vi "Photostimulation UI.vi"() -> ()   [LabVIEW 2012]
uses:
  GFG/GFGnumericGet.vi
  GFG/GFG library.lvlib
  <vilib>/vision/NI_Vision_Development_Module.lvlib
panel:
  out "deco string":string="Press and hold Ctrl to add multiple ROIs" caption="multiple points"
  in  "number of spots":dbl=5e-05 min=0.0 max=1.0 step=1.0 format="%#_6p"
  in  "Close":bool caption="QUIT"
  in  "spot repetitions":dbl=1.0 min=1.0 step=1.0
  out "error out":errorcluster
  in  "stop":bool
  in  "wait for external trigger":bool
  in  "stim duration (in seconds)":dbl=5e-05 caption="10us to 2ms" min=1e-05 max=0.002 step=1e-05 format="%#_6p"
  in  "pre-stim settling time (in seconds)":dbl=5e-05 caption="0 to 1s" min=0.0 max=1.0 step=0.0001 format="%#_6p"
  in  "stim interval (in seconds)":dbl=5e-05 caption="50us to 1s" min=5e-05 max=1.0 step=0.005 format="%#_6p"
  in  "group repetitions":dbl=1.0 min=1.0 step=1.0
  in  "stim power (%)":dbl(slide) scale=0.0..100.0
  out "Image":T1(plugin-control)
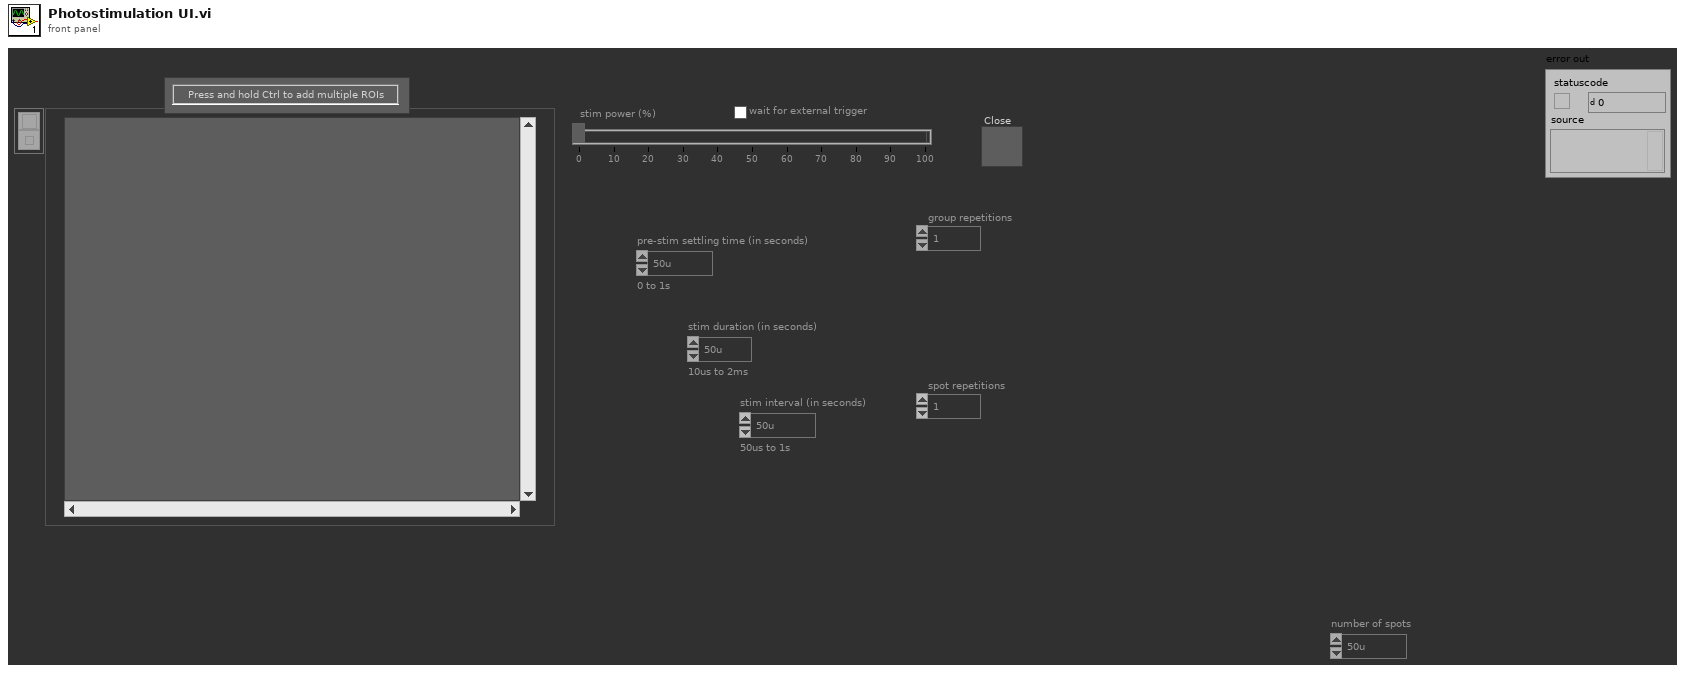
[diagram p1: front panel]
types:
  T1 = typedef "IMAQ Image.ctl" = refnum<image>
  T2 = cluster{"Global Rectangle":i32[], "Contours":cluster{"Contour Type":u32, "ROI Type":u32, "Points":i32[]}[]}
  T3 = typedef "Image Type" = u32
  T4 = cluster{"pre-stim settling time (in seconds)":dbl, "stim duration (in seconds)":dbl, "stim interval (in seconds)":dbl, "spot repetitions":dbl, "group repetitions":dbl, "number of spots":dbl}
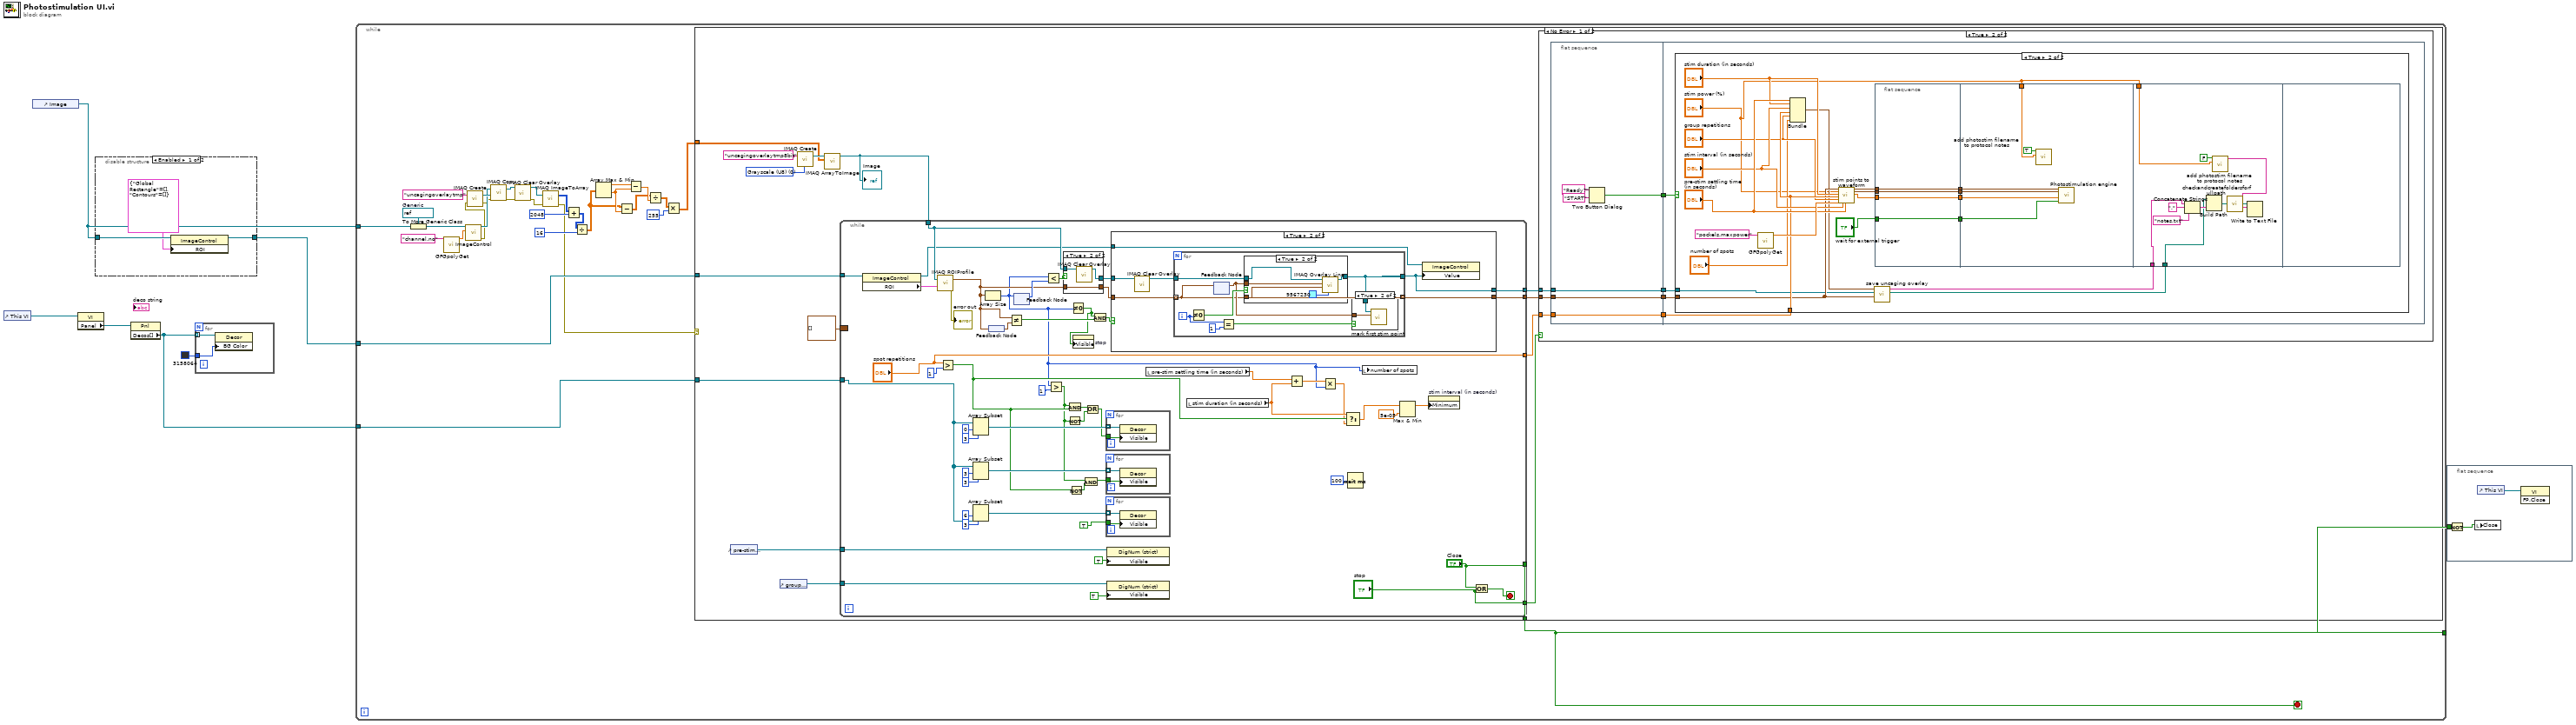
[diagram p0: block diagram]
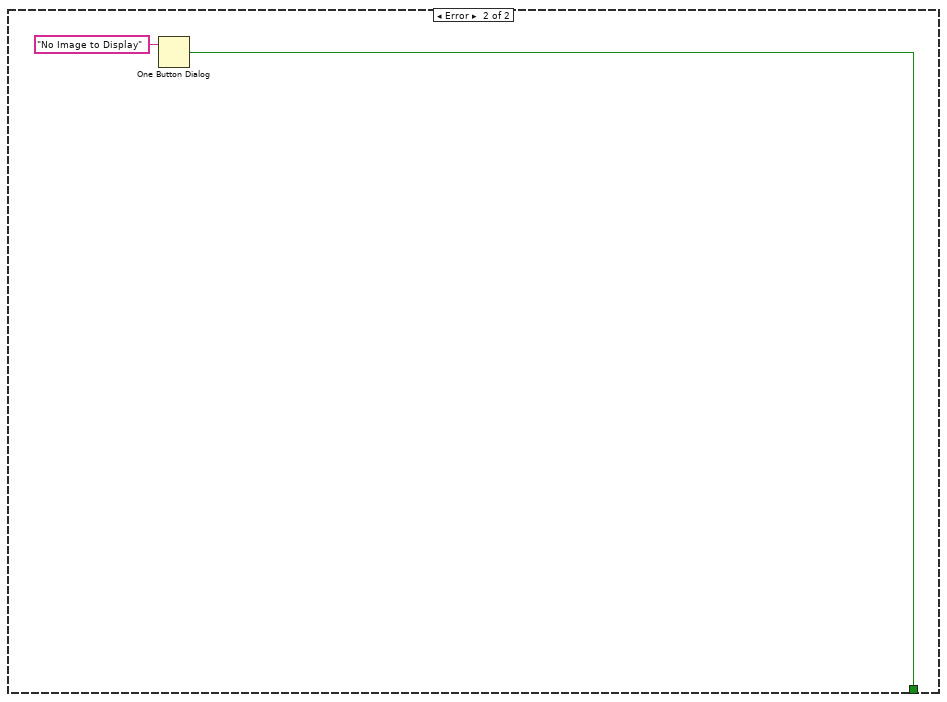
[diagram p8: hidden frame]
diagram:
  n1 = control-ref of="This VI"() -> (w7:refnum<vi>)
  n2 = control-ref of="Image"() -> (w3:refnum<vi>)
  n3 = property class="VI"(reference=w7) -> ("Panel"=w6:refnum<vi>)  [unwired: 1 in, 2 out]
  n4 = disable-structure shown="Enabled" {
    disable-tunnel: w3 -> [w10 w11]
    disable-tunnel: [w8 w11] -> w2
    frame Enabled {
      n5 = property class="ImageControl"(reference=w10, "ROI"=T2 {"Global Rectangle"=[], "Contours"=[]}) -> (reference out=w8:refnum<vi>)  [unwired: 1 in, 1 out]
    }
    frame Disabled {
    }
  }
  n6 = property class="Pnl"(reference=w6) -> ("Decos[]"=w5:refnum<vi>[])  [unwired: 1 in, 2 out]
  n7 = for {
    tunnel: w5 -> [w13] mode=indexing
    tunnel: u32 3158064 ("Color") -> [w12]
    n8 = property class="Decor"(reference=w13, "BG Color"=w12) -> ()  [unwired: 1 in, 2 out]
  }
  n9 = while {
    tunnel: w5 -> [w22]
    tunnel: w3 -> [w21]
    tunnel: w2 -> [w20]
    tunnel: [w19] -> w1
    stop <- w19 stop-if-true
    w43 = refnum<vi> refnum  # Generic
    n10 = To More Generic Class(target class=w43, reference=w21) -> (generic class reference=w42:refnum<vi>)
    n11 = call-poly "GFGpolyGet.vi"("Variable Name in"="channel.no") -> ("Numeric"=w41:dbl)  [unwired: 8 in, 2 out]
    n12 = call "ImageControl.vi"("Channel No"=w41, "Image Refnum (Generic)"=w42) -> ("Error Out"=w18:errorcluster, "Current Image"=w23:T1)  [unwired: 8 in]
    n13 = call "IMAQ Create"("Image Name"="uncagingoverlaytmp", "error in (no error)"=w18) -> ("New Image"=w38:T1, "error out"=w17:errorcluster)  [unwired: 3 in]
    n14 = call "IMAQ Copy"("error in (no error)"=w17, "Image Dst"=w38, "Image Src"=w23) -> ("error out"=w16:errorcluster, "Image Dst Out"=w37:T1)  [unwired: 3 in]
    n15 = call "IMAQ Clear Overlay"("error in (no error)"=w16, "Image"=w37) -> ("error out"=w15:errorcluster, "Image Out"=w36:T1)  [unwired: 8 in]
    n16 = call "IMAQ ImageToArray"("error in (no error)"=w15, "Image"=w36) -> ("error out"=w14:errorcluster, "Image Pixels (I16)"=w32:i16[][])  [unwired: 2 in, 3 out]
    n17 = Add(x=w32, y=i16 2048 ("index")) -> (x+y=w34:i16[][])
    n18 = Divide(x=w34, y=i16 16 ("index")) -> (x/y=w29:dbl[][])
    n19 = Array Max & Min(array=w29) -> (max value=w31:dbl, min value=w30:dbl)  [unwired: 2 out]
    n20 = Subtract(x=w29, y=w30) -> (x-y=w27:dbl[][])
    n21 = Subtract(x=w31, y=w30) -> (x-y=w28:dbl)
    n22 = Divide(x=w27, y=w28) -> (x/y=w26:dbl[][])
    n23 = Multiply(x=w26, y=i16 255 ("index")) -> (x*y=w25:dbl[][])
    n24 = case shown="No Error" w14 {
      tunnel: w25 -> [w55 _]
      tunnel: w22 -> [w52 _]
      tunnel: w20 -> [w50 _]
      tunnel: [w45 w206] -> w19
      frame No Error {
        w57 = T3 0 items=["Grayscale (U8)", "Grayscale (I16)", "Grayscale (SGL)", "Complex (CSG)", "RGB (U32)", "HSL (U32)", "RGB (U64)", "Grayscale (U16)"] ("Image Type")
        n25 = control-ref of="pre-stim settling time (in seconds)"() -> (w53:refnum<vi>)
        n26 = control-ref of="group repetitions"() -> (w51:refnum<vi>)
        n27 = call "IMAQ Create"("Image Name"="uncagingoverlaytmp8bit", "Image Type"=w57) -> ("New Image"=w56:T1)  [unwired: 3 in, 1 out]
        n28 = call "IMAQ ArrayToImage"("Image Pixels (U8)"=w55, "Image"=w56) -> ("Image Out"=w54:T1)  [unwired: 8 in, 1 out]
        "Image" <- w54
        n29 = while {
          tunnel: w50 -> [w111]
          tunnel: w54 -> [w105]
          tunnel: w52 -> [w86]
          tunnel: w53 -> [w99]
          tunnel: w51 -> [w89]
          tunnel: [w78] -> w49
          tunnel: ["spot repetitions"] -> w48
          tunnel: ["Close"] -> w45
          tunnel: [w65] -> w47
          tunnel: ["stop"] -> w46
          border: cluster{"X":u32, "Y":u32}[] [] ("Pixel Coordinates") -> [_]
          stop <- w67 stop-if-true
          n30 = property class="ImageControl"(reference=w111) -> (reference out=w102:refnum<vi>, "ROI"=w109:T2)  [unwired: 1 in, 1 out]
          n31 = call "IMAQ ROIProfile"("ROI Descriptor"=w109, "Image"=w105) -> ("error out"=→"error out":errorcluster, "Pixel Coordinates"=w81:cluster{"X":u32, "Y":u32}[])  [unwired: 2 in, 3 out]
          n32 = Greater?(x="spot repetitions", y=1) -> (0:w72:bool)
          n33 = Array Subset(array=w86, index=0, length=3) -> (w92:refnum<vi>[])
          n34 = Array Subset(array=w86, index=3, length=3) -> (w91:refnum<vi>[])
          n35 = Array Subset(array=w86, index=6, length=3) -> (w85:refnum<vi>[])
          n36 = Array Size(array=w81) -> (size(s)=w63:i32)
          n37 = feedback #1() -> (w82:cluster{"X":u32, "Y":u32}[])
          n38 = feedback-in #1(w81) -> ()
          n39 = Not Equal?(x=w81, y=w82) -> (x != y?=w108:bool)
          n40 = feedback-in #2(w63) -> ()
          n41 = feedback #2() -> (w107:i32)  [unwired: 1 in]
          n42 = Less?(x=w63, y=w107) -> (x < y?=w106:bool)
          n43 = Greater?(x=w63, y=1) -> (0:w71:bool)
          n44 = case shown="True" w106 {
            tunnel: w105 -> [w119 w122]
            tunnel: [w119 w121] -> w104
            tunnel: [w118 w120] -> w103
            tunnel: w81 -> [w118 w120]
            frame False {
            }
            frame True {
              n45 = call "IMAQ Clear Overlay"("Image"=w122) -> ("Image Out"=w121:T1)  [unwired: 9 in, 1 out]
            }
          }
          n46 = And(x=w71, y=w72) -> (x .and. y?=w90:bool)
          n47 = Not(x=w71) -> (.not. x?=w83:bool)
          n48 = Not(x=w72) -> (.not. x?=w79:bool)
          n49 = Not Equal To 0?(x=w63) -> (x != 0?=w62:bool)
          n50 = property on="stop" class="Bool"("Visible"=w62) -> ()  [unwired: 2 in, 2 out]
          n51 = And(x=w71, y=w79) -> (x .and. y?=w80:bool)
          n52 = Or(x=w90, y=w83) -> (x .or. y?=w84:bool)
          n53 = And(x=w62, y=w108) -> (x .and. y?=w98:bool)
          n54 = for {
            tunnel: w92 -> [w117] mode=indexing
            tunnel: w84 -> [w116]
            n55 = property class="Decor"(reference=w117, "Visible"=w116) -> ()  [unwired: 1 in, 2 out]
          }
          n56 = for {
            tunnel: w91 -> [w115] mode=indexing
            tunnel: w80 -> [w114]
            n57 = property class="Decor"(reference=w115, "Visible"=w114) -> ()  [unwired: 1 in, 2 out]
          }
          n58 = for {
            tunnel: w85 -> [w113] mode=indexing
            tunnel: TRUE -> [w112]
            n59 = property class="Decor"(reference=w113, "Visible"=w112) -> ()  [unwired: 1 in, 2 out]
          }
          n60 = property class="DigNum (strict)"(reference=w99, "Visible"=TRUE) -> ()  [unwired: 1 in, 2 out]
          n61 = property class="DigNum (strict)"(reference=w89, "Visible"=TRUE) -> ()  [unwired: 1 in, 2 out]
          n62 = case shown="True" w98 {
            tunnel: w104 -> [w123 w128]
            tunnel: w103 -> [w124 w130]
            tunnel: w102 -> [_ w129]
            tunnel: [w124 w126] -> w78
            tunnel: [w123 w125] -> w65
            frame False {
            }
            frame True {
              n63 = call "IMAQ Clear Overlay"("Image"=w128) -> ("Image Out"=w127:T1)  [unwired: 9 in, 1 out]
              n64 = for {
                tunnel: w130 -> [w131] mode=indexing
                tunnel: [w131] -> w126 mode=indexing
                tunnel: w127 -> [w138]
                tunnel: [w132] -> w125
                i -> [w136]
                n65 = Not Equal To 0?(x=w136) -> (x != 0?=w137:bool)
                n66 = feedback #3() -> (w133:cluster{"X":u32, "Y":u32})  [unwired: 1 in]
                n67 = feedback-in #3(w131) -> ()
                n68 = Equal?(x=w136, y=1) -> (x = y?=w134:bool)
                n69 = case shown="True" w137 {
                  tunnel: w138 -> [w141 w142]
                  tunnel: w133 -> [_ w146]
                  tunnel: w131 -> [_ w145]
                  tunnel: [w141 w144] -> w132
                  frame False {
                  }
                  frame True {
                    n70 = call "IMAQ Overlay Line"("Color"=u32 9567230, "End Point"=w145, "Start Point"=w146, "Image"=w142) -> ("Image Out"=w144:T1)  [unwired: 6 in, 1 out]
                  }
                }
                n71 = case shown="True" w134 {
                  tunnel: w133 -> [_ w140]
                  tunnel: w132 -> [_ w139]
                  frame False {
                  }
                  frame True {
                    n72 = call "mark first stim point.vi"("pixel coordinate"=w140, "Image In"=w139) -> ()  [unwired: 10 in]
                  }
                }
              }
              n73 = property class="ImageControl"(reference=w129, "Value"=w125) -> ()  [unwired: 1 in, 2 out]
            }
          }
          n74 = local read "pre-stim settling time (in seconds)"() -> (w74:dbl)
          n75 = local read "stim duration (in seconds)"() -> (w73:dbl)
          n76 = Add(x=w74, y=w73) -> (x+y=w70:dbl)
          n77 = Multiply(x=w70, y=w63) -> (x*y=w69:dbl)
          n78 = Select(t=w73, s=w72, f=w69) -> (s? t:f=w68:dbl)
          n79 = Wait (ms)(milliseconds to wait=u32 100) -> ()  [unwired: 1 out]
          n80 = local write "number of spots"(w63) -> ()
          n81 = Max & Min(x=w68, y=5e-05 ("Data Entry Limits:Minimum")) -> (max(x,y)=w75:dbl)  [unwired: 1 out]
          n82 = property on="stim interval (in seconds)" class="DigNum (strict)"("Minimum"=w75) -> ()  [unwired: 2 in, 2 out]
          n83 = Or(x="Close", y="stop") -> (x .or. y?=w67:bool)
        }
        n84 = case shown="True" w46 {
          tunnel: w49 -> [_ w150]
          tunnel: w48 -> [_ w149]
          tunnel: w47 -> [_ w147]
          frame False {
          }
          frame True {
            n85 = flat-sequence {
              tunnel: w149 -> [w158]
              tunnel: w150 -> [w159]
              tunnel: [w159] -> w153
              tunnel: [w158] -> w152
              tunnel: [w157] -> w151
              tunnel: [w154] -> w148
              tunnel: w147 -> [w154]
              tunnel: w153 -> [w163]
              tunnel: w152 -> [w162]
              tunnel: w151 -> [w161]
              tunnel: w148 -> [w160]
              frame #0 {
                n86 = Two Button Dialog(message="Ready?", 2:"START" ("T button name (\"OK\")")) -> (T button?=w157:bool)  [unwired: 1 in]
              }
              frame #1 {
                n87 = case shown="True" w161 {
                  tunnel: w163 -> [_ w173]
                  tunnel: w162 -> [_ w176]
                  tunnel: w160 -> [_ w172]
                  frame False {
                  }
                  frame True {
                    n88 = call-poly "GFGpolyGet.vi"("Variable Name in"="pockels.maxpower") -> ("Numeric"=w184:dbl)  [unwired: 8 in, 2 out]
                    n89 = Bundle("pre-stim settling time (in seconds)"="pre-stim settling time (in seconds)", "stim duration (in seconds)"="stim duration (in seconds)", "stim interval (in seconds)"="stim interval (in seconds)", "spot repetitions"=w176, "group repetitions"="group repetitions", "number of spots"="number of spots") -> (w171:T4)  [unwired: 1 in]
                    n90 = call "stim points to waveform.vi"("stim point array"=w173, "stim power (%)"="stim power (%)", "stim duration (in seconds)"="stim duration (in seconds)", "spot repetitions"=w176, "group repetitions"="group repetitions", "pockels cell max power"=w184, "stim interval (in seconds)"="stim interval (in seconds)", "pre-stim settling time (in seconds)"="pre-stim settling time (in seconds)") -> ("x-y mirror data out"=w183:waveform(dbl)[], "pockels and piezo data out"=w182:waveform(dbl)[], "repetitions"=w181:dbl)  [unwired: 9 in]
                    n91 = call "save uncaging overlay.vi"("Pixel Coordinates"=w173, "Image"=w172, "param cluster"=w171) -> ("stripped path"=w169:path, "filename without extension"=w170:string)  [unwired: 7 in]
                    n92 = flat-sequence {
                      tunnel: "wait for external trigger" -> [w186]
                      tunnel: w181 -> [w187]
                      tunnel: w182 -> [w188]
                      tunnel: w183 -> [w189]
                      tunnel: [w189] -> w168
                      tunnel: [w188] -> w167
                      tunnel: [w187] -> w166
                      tunnel: [w186] -> w165
                      tunnel: w168 -> [w195]
                      tunnel: w167 -> [w194]
                      tunnel: w166 -> [w193]
                      tunnel: w165 -> [w192]
                      tunnel: "stim power (%)" -> [w190]
                      tunnel: w170 -> [w198]
                      tunnel: w169 -> [w199]
                      tunnel: "stim power (%)" -> [w196]
                      frame #0 {
                      }
                      frame #1 {
                        n93 = call "add photostim filename to protocol notes.vi"("stim power"=w190, "rec start/end (T is start)"=TRUE) -> ()  [unwired: 9 in, 1 out]
                        n94 = call "Photostimulation engine.vi"("external trigger enabled?"=w192, "waveform repetitions"=w193, "pockels and piezo data in"=w194, "x-y mirror data in"=w195) -> ()  [unwired: 8 in]
                      }
                      frame #2 {
                        n95 = Concatenate Strings(w198, "." ("string"), "notes.txt" ("string")) -> (w203:string)
                        n96 = Build Path(base path=w199, name or relative path=w203) -> (appended path=w200:path)
                        n97 = call "add photostim filename to protocol notes.vi"("stim power"=w196, "rec start/end (T is start)"=FALSE) -> ("protocol.notes out"=w197:string)  [unwired: 9 in]
                        n98 = call "checkandcreatefoldersforfullpath.vi"("Path IN"=w200) -> ("Path OUT"=w204:path)  [unwired: 4 in]
                        n99 = Write to Text File(file (use dialog)=w204, text=w197) -> ()  [unwired: 2 in, 3 out]
                      }
                      frame #3 {
                      }
                    }
                  }
                }
              }
            }
          }
        }
      }
      frame Error {
        n100 = One Button Dialog(message="No Image to Display") -> (true=w206:bool)  [unwired: 1 in]
      }
    }
  }
  n101 = flat-sequence {
    tunnel: w1 -> [w210]
    frame #0 {
      n102 = Not(x=w210) -> (.not. x?=w209:bool)
      n103 = local write "Close"(w209) -> ()
      n104 = control-ref of="This VI"() -> (w208:refnum<vi>)
      n105 = invoke class="VI" method="FP.Close"(reference=w208) -> ()  [unwired: 2 in, 3 out]
    }
  }
